vi "TDMS引用.vi"() -> ()   [LabVIEW 2020]
panel:
  in  "组名称":string
  out "tdms文件":refnum<k34>
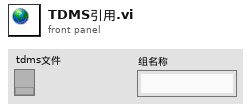
[diagram p1: front panel]
diagram:
